vi "扭矩模式.vi"(8 "error in (no error)":errorcluster, 10 "Max Torque":sgl=9.0) -> (0 "error out":errorcluster)   [LabVIEW 2020, in "输出轴伺服.lvlib"]
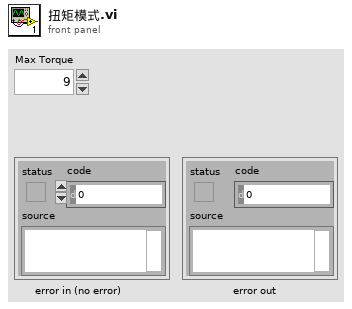
[diagram p1: front panel]
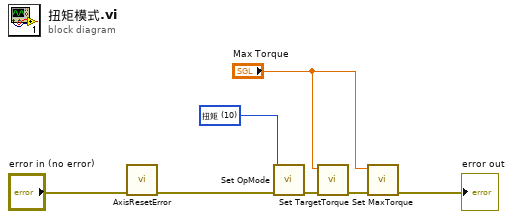
[diagram p0: block diagram]
diagram:
  w3 = u32 10 items=["位移"=8, "速度"=9, "扭矩"=10] ("Value")
  n1 = call "AxisResetError.vi"("error in (no error)"="error in (no error)") -> ("error out"=w2:errorcluster)  [unwired: 10 in]
  n2 = call "Set OpMode.vi"("error in (no error)"=w2, "Value"=w3) -> ("error out"=w7:errorcluster)  [unwired: 9 in]
  n3 = call "Set TargetTorque.vi"("error in (no error)"=w7, "Value"="Max Torque") -> ("error out"=w6:errorcluster)  [unwired: 9 in]
  n4 = call "Set MaxTorque.vi"("error in (no error)"=w6, "Value"="Max Torque") -> ("error out"=→"error out":errorcluster)  [unwired: 9 in]
